vi "FindLibPath.vi"(10 "Caraya Library Member Path":path) -> (2 "Caraya Library Path":path)   [LabVIEW 2013, in "Caraya.lvlib"]
uses:
  Caraya.lvlib
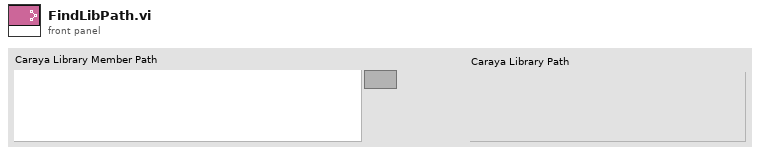
[diagram p1: front panel]
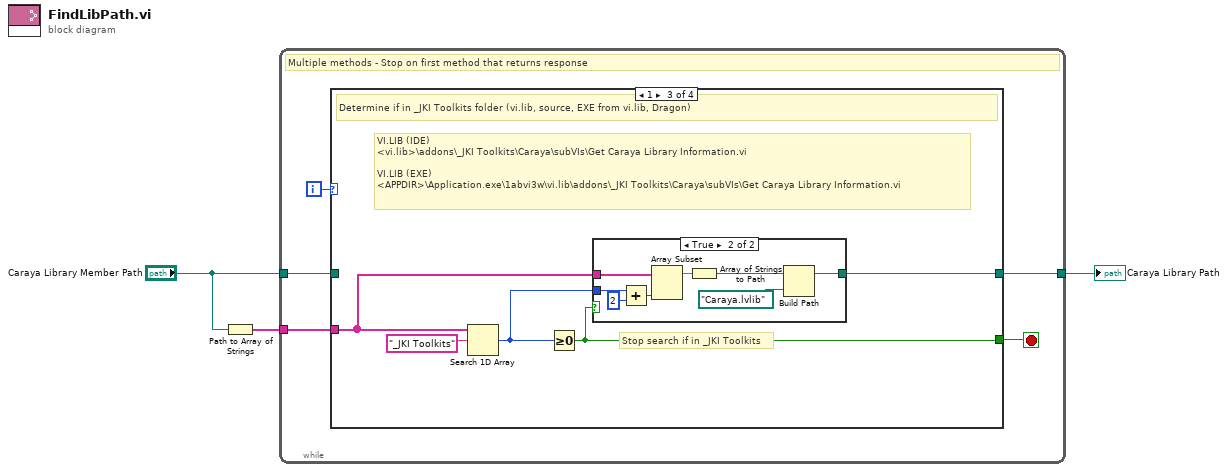
[diagram p0: block diagram]
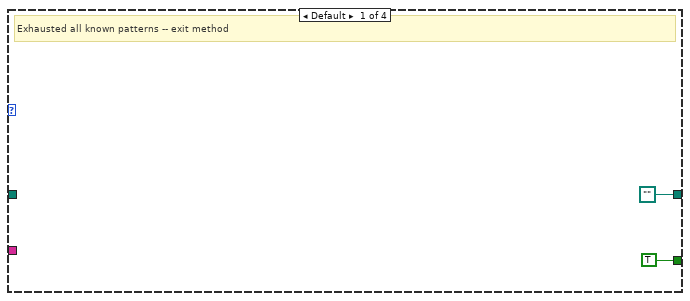
[diagram p2: hidden frame]
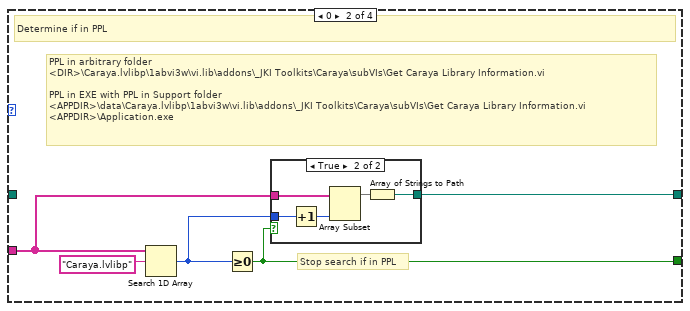
[diagram p3: hidden frame]
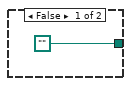
[diagram p4: hidden frame]
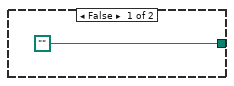
[diagram p5: hidden frame]
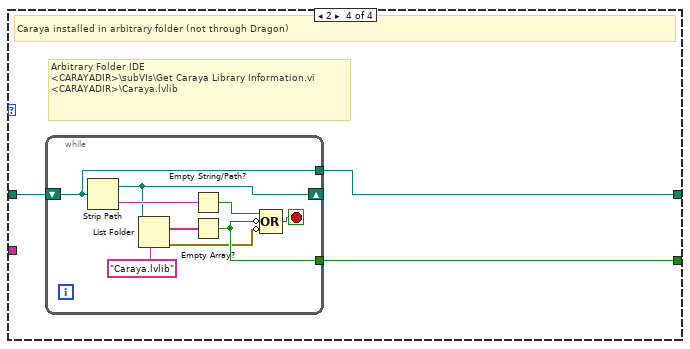
[diagram p6: hidden frame]
diagram:
  n1 = Path to Array of Strings(0:"Caraya Library Member Path") -> (2:w1:string[])  [unwired: 1 out]
  n2 = while {
    tunnel: "Caraya Library Member Path" -> [w8]
    tunnel: [w7] -> w2
    tunnel: w1 -> [w6]
    i -> [w5]
    stop <- w4 stop-if-true
    # "Multiple methods - Stop on first method that returns response"
    n3 = case shown="1" w5 {
      tunnel: w8 -> [_ _ _ w38]
      tunnel: [path "" w13 w24 w37] -> w7
      tunnel: w6 -> [_ w12 w23 _]
      tunnel: [TRUE w11 w22 w36] -> w4
      frame Default {
        # "Exhausted all known patterns -- exit method"
      }
      frame 0 {
        # "PPL in arbitrary folder\n<DIR>\\Caraya.lvlibp\\1abvi3w\\vi.lib\\addons\\_JKI Toolkits\\Caraya\\subVIs\\Get Caraya Library Information.vi\n\nPPL in EXE with PPL in Support folder\n<APPDIR>\\data\\Caraya.lvlibp\\1abvi3w\\vi.lib\\addons\\_JKI Toolkits\\Caraya\\subVIs\\Get Caraya Library Information.vi\n<APPDIR>\\Application.exe"
        # "Stop search if in PPL"
        # "Determine if in PPL"
        n4 = Search 1D Array(1D array=w12, element="Caraya.lvlibp" ("y")) -> (index of element=w14:i32)  [unwired: 1 in]
        n5 = Greater Or Equal To 0?(x=w14) -> (x >= 0?=w11:bool)
        n6 = case shown="True" w11 {
          tunnel: w14 -> [_ w21]
          tunnel: [path "" w20] -> w13
          tunnel: w12 -> [_ w17]
          frame False {
          }
          frame True {
            n7 = Increment(x=w21) -> (x+1=w18:i32)
            n8 = Array Subset(array=w17, length=w18) -> (w19:string[])  [unwired: 1 in]
            n9 = Array of Strings to Path(0:w19) -> (2:w20:path)  [unwired: 1 in]
          }
        }
      }
      frame 1 {
        # "VI.LIB (IDE)\n<vi.lib>\\addons\\_JKI Toolkits\\Caraya\\subVIs\\Get Caraya Library Information.vi\n\nVI.LIB (EXE)\n<APPDIR>\\Application.exe\\1abvi3w\\vi.lib\\addons\\_JKI Toolkits\\Caraya\\subVIs\\Get Caraya Library Information.vi"
        # "Stop search if in _JKI Toolkits"
        # "Determine if in _JKI Toolkits folder (vi.lib, source, EXE from vi.lib, Dragon)"
        n10 = Search 1D Array(1D array=w23, element="_JKI Toolkits" ("y")) -> (index of element=w25:i32)  [unwired: 1 in]
        n11 = Greater Or Equal To 0?(x=w25) -> (x >= 0?=w22:bool)
        n12 = case shown="True" w22 {
          tunnel: w25 -> [_ w32]
          tunnel: [path "" w28] -> w24
          tunnel: w23 -> [_ w33]
          frame False {
          }
          frame True {
            n13 = Add(x=w32, y=2) -> (x+y=w34:i32)
            n14 = Array Subset(array=w33, length=w34) -> (w35:string[])  [unwired: 1 in]
            n15 = Array of Strings to Path(0:w35) -> (2:w29:path)  [unwired: 1 in]
            n16 = Build Path(base path=w29, name or relative path=path "Caraya.lvlib") -> (appended path=w28:path)
          }
        }
      }
      frame 2 {
        # "Arbitrary Folder IDE\n<CARAYADIR>\\subVIs\\Get Caraya Library Information.vi\n<CARAYADIR>\\Caraya.lvlib"
        # "Caraya installed in arbitrary folder (not through Dragon)"
        n17 = while {
          shift-right: [w43] -> _
          shift-left: w38 -> [w45]
          tunnel: [w45] -> w37
          tunnel: [w40] -> w36
          stop <- w44 stop-if-true
          n18 = Strip Path(path=w45) -> (stripped path=w43:path, name=w47:string)
          n19 = List Folder(path=w43, pattern="Caraya.lvlib" ("y")) -> (filenames=w41:string[], error out=w39:errorcluster)  [unwired: 2 in, 2 out]
          n20 = Empty String/Path?(string/path=w47) -> (empty?=w46:bool)
          n21 = Empty Array?(array=w41) -> (empty?=w40:bool)
          n22 = Compound Arithmetic op=OR(w46, invert w40, invert w39) -> (w44:bool)
        }
      }
    }
  }
  "Caraya Library Path" <- w2
